vi "Layout - CSV quoting.vi"(8 "error in (no error)":errorcluster) -> (0 "error out":errorcluster)   [LabVIEW 2026, in "Tests.lvlib"]
doc: "Unit test (Caraya). Verifies CSVQuoteField applies RFC 4180 quoting: a plain field is unquoted; a field containing a double quote, the configured delimiter, or a newline is wrapped in quotes with internal quotes doubled; and quoting is evaluated against the configured delimiter, not a fixed comma (SRS-LMBR-012). Pure string-in/string-out, no fixtures."
uses:
  Tests.lvlib
  <vilib>/addons/_JKI Toolkits/Caraya/classes/Assert/Assert Equal Value_Variant.vi
  <vilib>/addons/_JKI Toolkits/Caraya/classes/Assert/Assert.lvclass
  <vilib>/addons/_JKI Toolkits/Caraya/classes/Test/Test.lvclass
  src/Lumberjack.lvlib
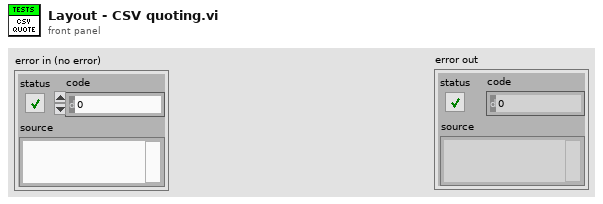
[diagram p1: front panel]
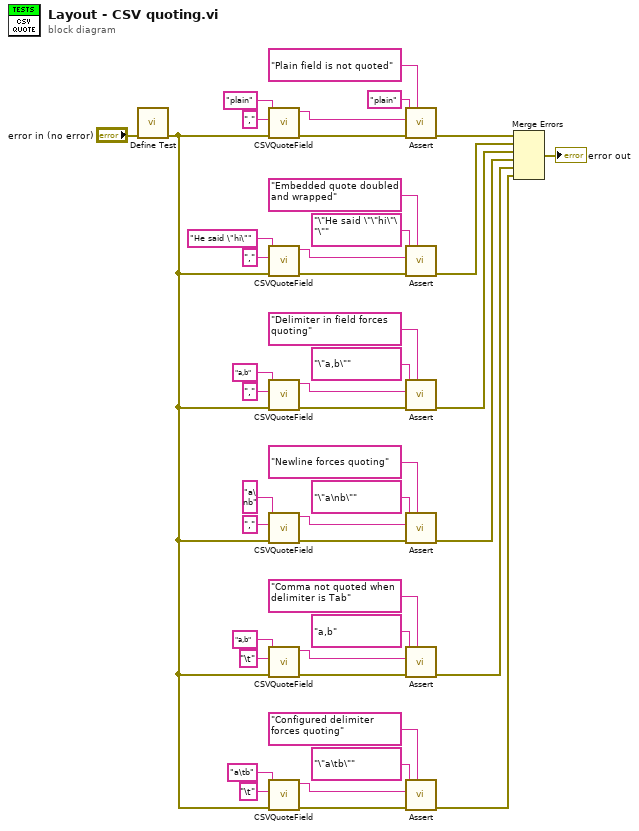
[diagram p0: block diagram]
diagram:
  n1 = call <vilib>:"Define Test.vi"("error in (no error)"="error in (no error)") -> ("error out"=w1:errorcluster)  [unwired: 9 in, 1 out]
  n2 = call "CSVQuoteField.vi"("error in (no error)"=w1, "delimiter"=",", "field"="plain" ("message")) -> ("error out"=w43:errorcluster, "quotedField"=w40:string)  [unwired: 7 in]
  n3 = call "CSVQuoteField.vi"("error in (no error)"=w1, "delimiter"=",", "field"="He said \"hi\"" ("message")) -> ("error out"=w37:errorcluster, "quotedField"=w34:string)  [unwired: 7 in]
  n4 = call "CSVQuoteField.vi"("error in (no error)"=w1, "delimiter"=",", "field"="a,b" ("message")) -> ("error out"=w28:errorcluster, "quotedField"=w25:string)  [unwired: 7 in]
  n5 = call "CSVQuoteField.vi"("error in (no error)"=w1, "delimiter"=",", "field"="a\nb" ("message")) -> ("error out"=w21:errorcluster, "quotedField"=w18:string)  [unwired: 7 in]
  n6 = call "CSVQuoteField.vi"("error in (no error)"=w1, "delimiter"="\t", "field"="a,b" ("message")) -> ("error out"=w14:errorcluster, "quotedField"=w11:string)  [unwired: 7 in]
  n7 = call "CSVQuoteField.vi"("error in (no error)"=w1, "delimiter"="\t", "field"="a\tb" ("message")) -> ("error out"=w8:errorcluster, "quotedField"=w5:string)  [unwired: 7 in]
  n8 = call-poly <vilib>:"Assert.vi"("Label"="Plain field is not quoted", "error in (no error)"=w43, "Actual"=w40, "Expected"="plain" ("message")) -> ("error out"=w31:errorcluster)  [unwired: 6 in, 1 out]
  n9 = call-poly <vilib>:"Assert.vi"("Label"="Embedded quote doubled and wrapped", "error in (no error)"=w37, "Actual"=w34, "Expected"="\"He said \"\"hi\"\"\"" ("message")) -> ("error out"=w32:errorcluster)  [unwired: 6 in, 1 out]
  n10 = call-poly <vilib>:"Assert.vi"("Label"="Delimiter in field forces quoting", "error in (no error)"=w28, "Actual"=w25, "Expected"="\"a,b\"" ("message")) -> ("error out"=w23:errorcluster)  [unwired: 6 in, 1 out]
  n11 = call-poly <vilib>:"Assert.vi"("Label"="Newline forces quoting", "error in (no error)"=w21, "Actual"=w18, "Expected"="\"a\nb\"" ("message")) -> ("error out"=w16:errorcluster)  [unwired: 6 in, 1 out]
  n12 = call-poly <vilib>:"Assert.vi"("Label"="Comma not quoted when delimiter is Tab", "error in (no error)"=w14, "Actual"=w11, "Expected"="a,b" ("message")) -> ("error out"=w3:errorcluster)  [unwired: 6 in, 1 out]
  n13 = call-poly <vilib>:"Assert.vi"("Label"="Configured delimiter forces quoting", "error in (no error)"=w8, "Actual"=w5, "Expected"="\"a\tb\"" ("message")) -> ("error out"=w2:errorcluster)  [unwired: 6 in, 1 out]
  n14 = Merge Errors(w31, w32, w23, w16, w3, w2) -> (→"error out":errorcluster)
